vi "Tip template creation and matching.vi"() -> ()   [LabVIEW 2018]
uses:
  <vilib>/userdefined/High Color/IMAQdx.ctl
  <vilib>/vision/driver/NI_Vision_Acquisition_Software.lvlib
  <vilib>/vision/NI_Vision_Development_Module.lvlib
panel:
  out "Image 3":T1(plugin-control)
  in  "搜索模板":bool
  in  "创建模板":bool
  out "Matches 2":T2(array[cluster]) {"Bounding Box"."y" format="%.2f"; "Bounding Box"."x" format="%.2f"; "Position"."y" format="%.2f"; "Position"."x" format="%.2f"; "Score" format="%.2f"; "Scale" format="%.2f"; "Angle" format="%.2f"}
  in  "Number of Matches Requested":i32=1 min=1
  in  "Minimum Match Score":sgl=300.0 min=0 max=1000 format="%.2f"
  in  "Match Mode":u16(ring) items=["Shift Invariant", "Rotation Invariant"]
  in  "Minimum Contrast":i32 min=0 max=255 step=1
  out "Number of Matches":i32
  in  "停止":bool
  out "Image 2":T1(plugin-control)
  out "Image":T1(plugin-control)
  in  "基路径":path
  in  "Session In":T3="cam1"
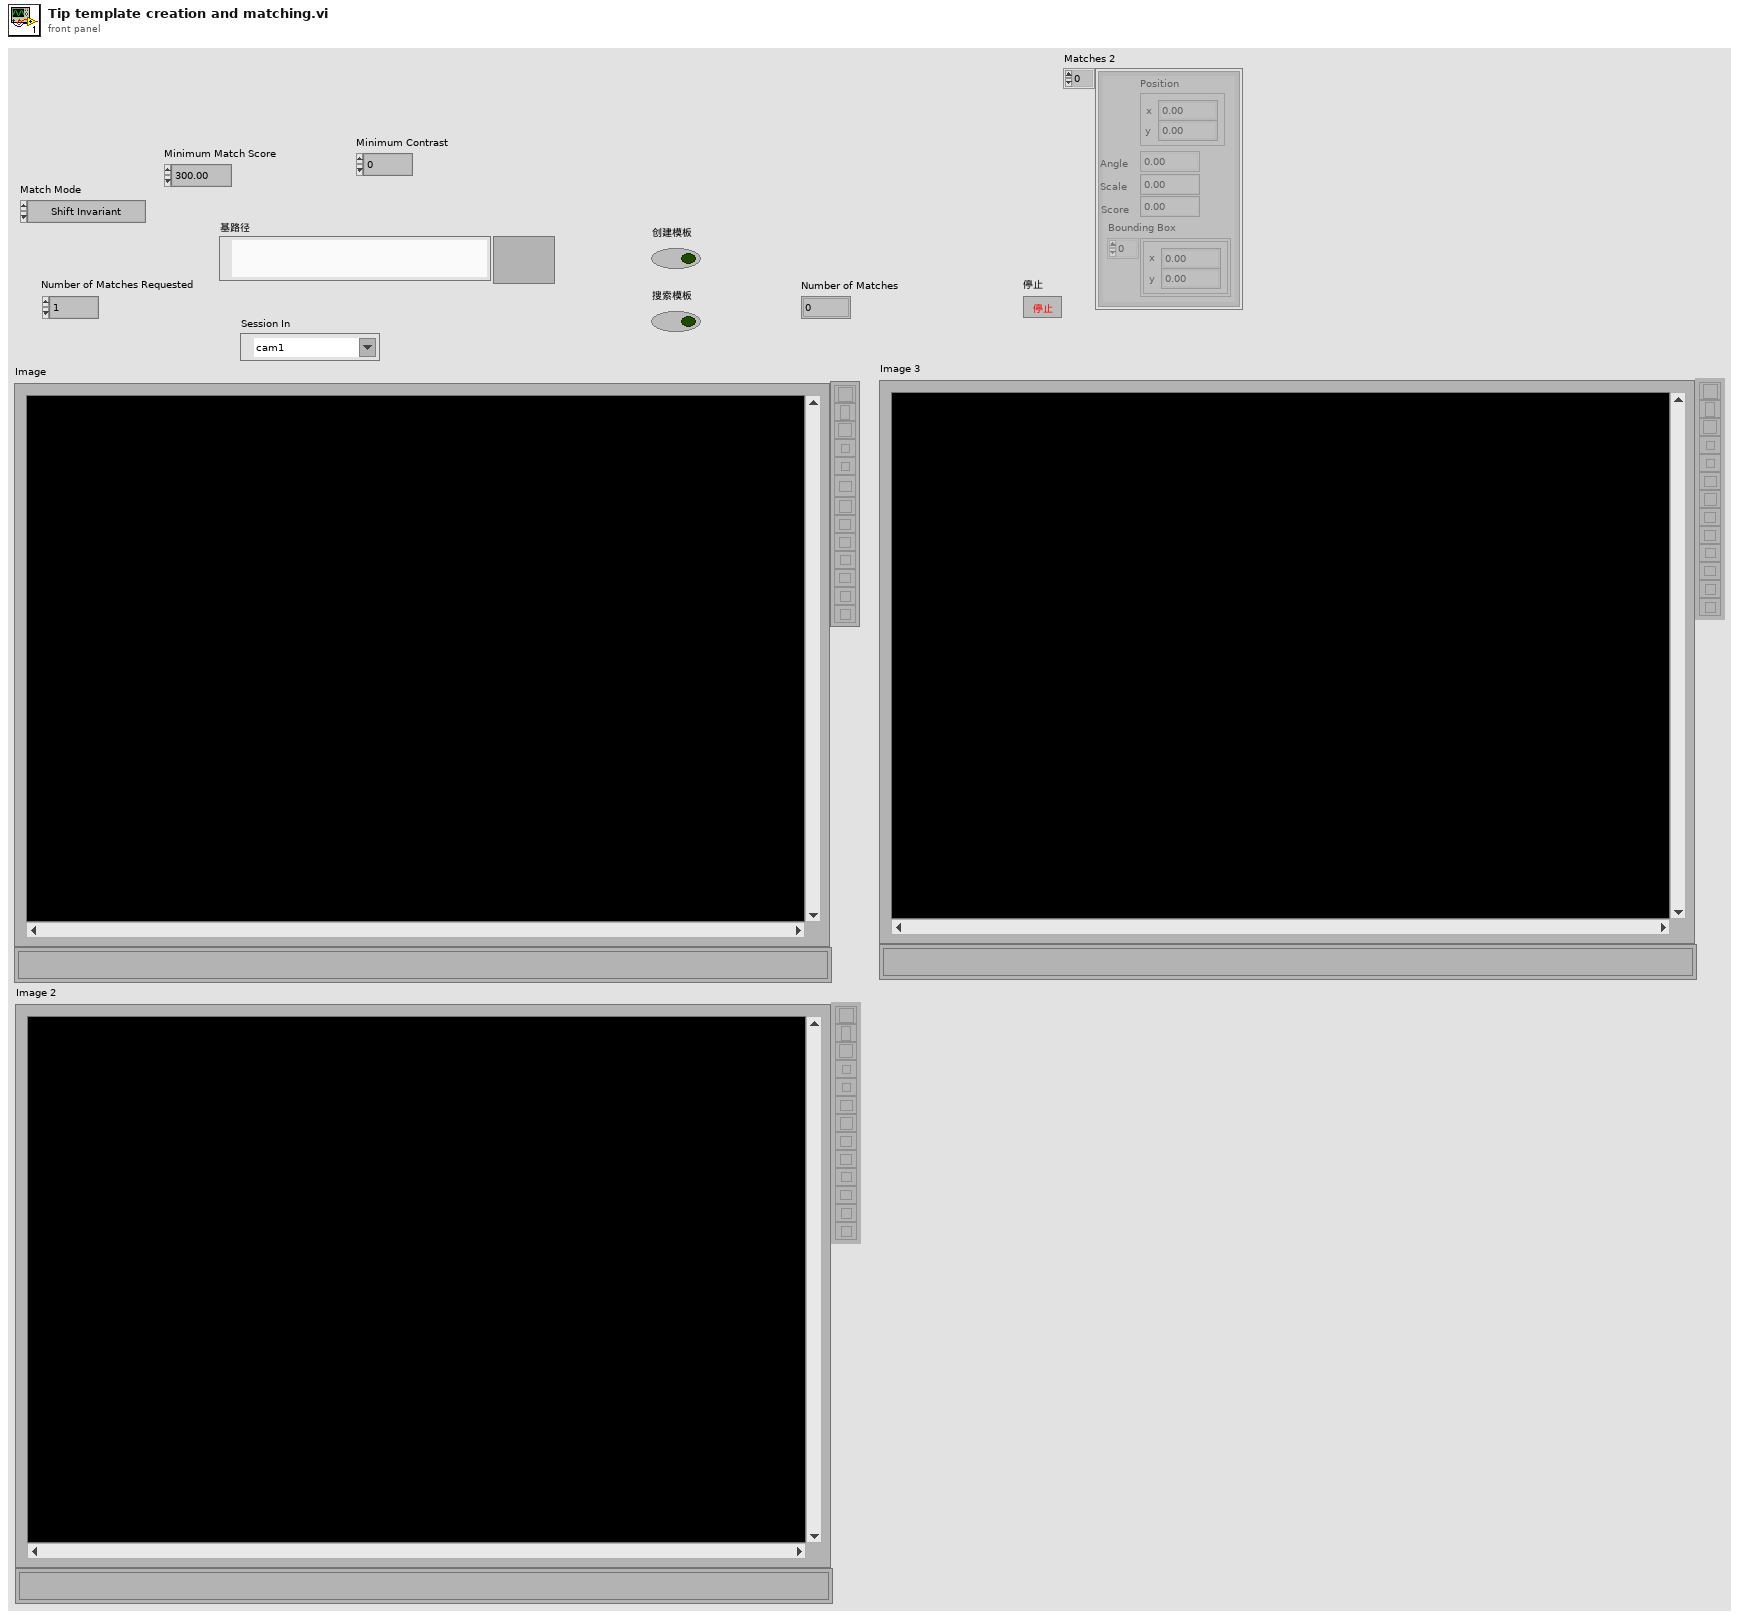
[diagram p1: front panel]
types:
  T1 = typedef "IMAQ Image.ctl" = refnum<image>
  T2 = cluster{"Position":cluster{"x":sgl, "y":sgl}, "Angle":sgl, "Scale":sgl, "Score":sgl, "Bounding Box":cluster{"x":sgl, "y":sgl}[]}[]
  T3 = typedef "IMAQdx.ctl" = refnum<k21>
  T4 = cluster{"Global Rectangle":i32[], "Contours":cluster{"Contour Type":u32, "ROI Type":u32, "Points":i32[]}[]}
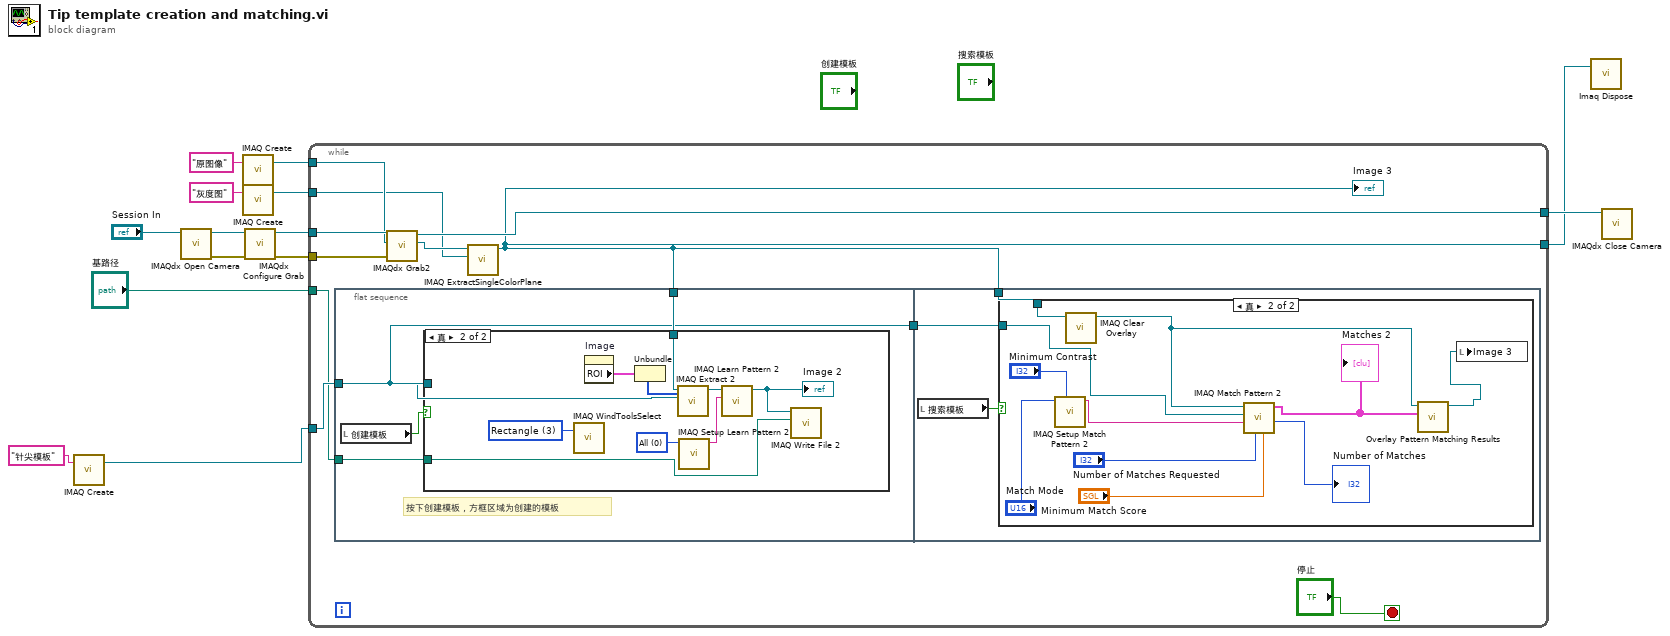
[diagram p0: block diagram]
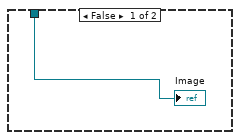
[diagram p3: hidden frame]
diagram:
  n1 = call "IMAQ Create"("Image Name"="针尖模板") -> ("New Image"=w4:T1)  [unwired: 4 in, 1 out]
  n2 = call <vilib>:"IMAQdx Open Camera.vi"("Session In"="Session In") -> ("error out"=w14:errorcluster, "Session Out"=w13:T3)  [unwired: 9 in]
  n3 = call "IMAQ Create"("Image Name"="原图像") -> ("New Image"=w8:T1)  [unwired: 4 in, 1 out]
  n4 = call "IMAQ Create"("Image Name"="灰度图") -> ("New Image"=w1:T1)  [unwired: 4 in, 1 out]
  n5 = call <vilib>:"IMAQdx Configure Grab.vi"("error in"=w14, "Session In"=w13) -> ("error out"=w10:errorcluster, "Session Out"=w11:T3)  [unwired: 8 in]
  n6 = while {
    tunnel: w11 -> [w25]
    tunnel: w10 -> [w24]
    tunnel: w8 -> [w23]
    tunnel: [w22] -> w7
    tunnel: [w15] -> w6
    tunnel: w4 -> [w20]
    tunnel: "基路径" -> [w18]
    tunnel: w1 -> [w16]
    stop <- "停止" stop-if-true
    n7 = flat-sequence {
      tunnel: w20 -> [w27]
      tunnel: w15 -> [w28]
      tunnel: [w27] -> w19
      tunnel: w18 -> [w26]
      tunnel: w15 -> [w42]
      tunnel: w19 -> [w40]
      frame #0 {
        # "按下创建模板，方框区域为创建的模板"
        n8 = local read "创建模板"() -> (w29:bool)
        n9 = case shown="真" w29 {
          tunnel: w27 -> [_ w33]
          tunnel: w28 -> [_ w32]
          tunnel: w26 -> [_ w30]
          frame False {
          }
          frame True {
            w38 = u32 3 items=["No Selection", "Point", "Line", "Rectangle", "Oval", "Polygon", "Freehand Region", "Annulus", "Zoom", "Pan", "Broken Line", "Freehand Line", "Rotated Rectangle"] ("Tool (Point)")
            w36 = u16 0 items=["All", "Shift Information", "Rotation Information"] ("Learn Mode")
            n10 = call "IMAQ WindToolsSelect"("Tool (Point)"=w38) -> ()  [unwired: 4 in, 2 out]
            n11 = property on="Image" class="ImageControl"() -> ("ROI"=w34:T4)  [unwired: 2 in, 2 out]
            n12 = Unbundle(w34) -> ("Global Rectangle"=w39:i32[])  [unwired: 1 out]
            n13 = call "IMAQ Extract 2"("Optional Rectangle"=w39, "Image Dst"=w33, "Image Src"=w32) -> ("Image Dst Out"=w37:T1)  [unwired: 7 in, 1 out]
            n14 = call "IMAQ Setup Learn Pattern 2"("Learn Mode"=w36) -> ("Learn Pattern Setup Data"=w35:string)  [unwired: 9 in, 1 out]
            n15 = call "IMAQ Learn Pattern 2"("Learn Pattern Setup Data"=w35, "Image"=w37) -> ("Template Image Out"=w31:T1)  [unwired: 8 in, 1 out]
            "Image 2" <- w31
            n16 = call-poly "IMAQ Write File 2"("File Path"=w30, "Image"=w31) -> ()  [unwired: 8 in, 2 out]
          }
        }
      }
      frame #1 {
        n17 = local read "搜索模板"() -> (w41:bool)
        n18 = case shown="真" w41 {
          tunnel: w42 -> [w43 w47]
          tunnel: w40 -> [_ w45]
          frame False {
            "Image" <- w43
          }
          frame True {
            n19 = call "IMAQ Setup Match Pattern 2"("Minimum Contrast"="Minimum Contrast", "Match Mode"="Match Mode") -> ("Match Pattern Setup Data"=w50:string)  [unwired: 8 in, 1 out]
            n20 = call "IMAQ Clear Overlay"("Image"=w47) -> ("Image Out"=w46:T1)  [unwired: 9 in, 1 out]
            n21 = call "IMAQ Match Pattern 2"("Minimum Match Score"="Minimum Match Score", "Number of Matches Requested"="Number of Matches Requested", "Match Pattern Setup Data"=w50, "Template Image"=w45, "Image"=w46) -> ("Number of Matches"=→"Number of Matches":i32, "Matches"=w54:T2)  [unwired: 4 in, 1 out]
            "Matches 2" <- w54
            n22 = call "Overlay Pattern Matching Results.vi"("Matches"=w54, "Image"=w46) -> ("Image Out"=w44:T1)  [unwired: 8 in, 1 out]
            n23 = local write "Image 3"(w44) -> ()
          }
        }
      }
    }
    n24 = call <vilib>:"IMAQdx Grab2.vi"("error in"=w24, "Image In"=w23, "Session In"=w25) -> ("Image Out"=w17:T1, "Session Out"=w22:T3)  [unwired: 5 in, 2 out]
    n25 = call "IMAQ ExtractSingleColorPlane"("Image Dst"=w16, "Image Src"=w17) -> ("Image Dst Out"=w15:T1)  [unwired: 8 in, 1 out]
    "Image 3" <- w15
  }
  n26 = call "Imaq Dispose"("Image"=w6) -> ()  [unwired: 5 in, 1 out]
  n27 = call <vilib>:"IMAQdx Close Camera.vi"("Session In"=w7) -> ()  [unwired: 10 in, 1 out]
